vi "Actor Core.vi"(8 "error in":errorcluster, 11 "CoolAppProcess in":refnum<class "CoolAppProcess.lvclass">) -> (0 "error out":errorcluster, 3 "Actor out":refnum<class "Actor.lvclass">)   [LabVIEW 2020, in "LAF2024Q2.lvlib" / "CoolAppProcess.lvclass"]
doc: "(<B>Filename</B>: Actor Framework.lvlib:Actor.lvclass:Actor Core.vi)\n\nReceives messages to the actor, reacts to them, and initiates any error handling that may shut the actor down.\n\nDescendant classes may override this VI to append parallel tasks for the actor to complete while it handles messages. Overrides use the Call Parent Class Method node."
uses:
  CoolAppProcess.lvclass
  C:/Program Files (x86)/National Instruments/LabVIEW 2020/vi.lib/ActorFramework/Actor/Actor.lvclass
  <vilib>/ActorFramework/Actor/Actor.lvclass
  Process State.ctl
  f1630098-5edb-487b-b4df-28bc80a2edd7.vi
  LAF2024Q2.lvlib
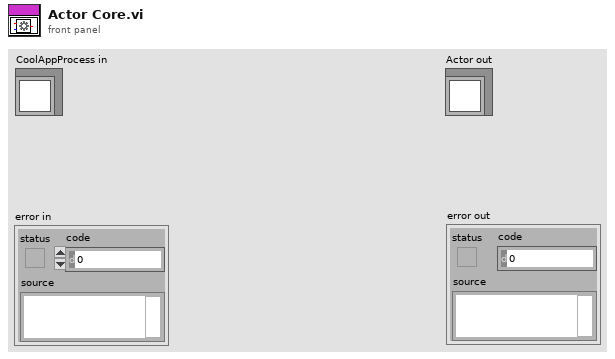
[diagram p1: front panel]
types:
  T1 = typedef "LAF2024Q2.lvlib/Process State.ctl" = enum16{"Idle", "Initializing", "Starting", "Running", "Stopping", "Stopped"}
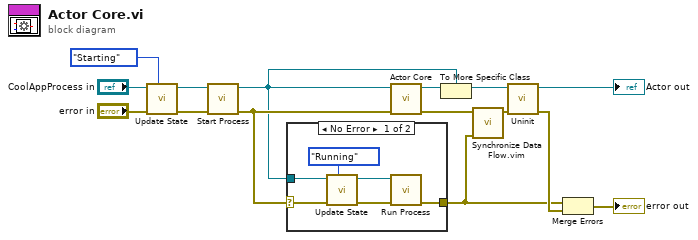
[diagram p0: block diagram]
diagram:
  n1 = call "Update State.vi"("Process State"=Process_State."Starting", "CoolAppProcess in"="CoolAppProcess in") -> ("CoolAppProcess out"=w5:refnum<class "CoolAppProcess.lvclass">)  [unwired: 9 in]
  n2 = call-dynamic "Start Process.vi"("error in (no error)"="error in", "CoolAppProcess in"=w5) -> ("error out"=w7:errorcluster, "CoolAppProcess out"=w6:refnum<class "CoolAppProcess.lvclass">)  [unwired: 8 in]
  n3 = case shown="No Error" w7 {
    selector: w7 -> [w19 _]
    tunnel: w6 -> [w18 _]
    tunnel: [w17 _] -> w1
    frame No Error {
      n4 = call "Update State.vi"("Process State"=Process_State."Running", "CoolAppProcess in"=w18) -> ("CoolAppProcess out"=w16:refnum<class "CoolAppProcess.lvclass">)  [unwired: 9 in]
      n5 = call-dynamic "Run Process.vi"("error in (no error)"=w19, "CoolAppProcess in"=w16) -> ("error out"=w17:errorcluster)  [unwired: 8 in, 1 out]
    }
    frame Error {
    }
  }
  n6 = call-parent "Actor Core.vi"("error in"=w7, "Actor in"=w6) -> ("error out"=w3:errorcluster, "Actor out"=w13:refnum<class "Actor.lvclass">)  [unwired: 8 in]
  n7 = To More Specific Class(target class=w6, reference=w13) -> (specific class reference=w11:refnum<class "CoolAppProcess.lvclass">)  [unwired: 1 in, 1 out]
  n8 = call "Synchronize Data Flow.vim"("input 4"=w1, "input 1"=w3) -> ("output 1"=w2:errorcluster)  [unwired: 2 in, 3 out]
  n9 = call "Uninit.vi"("error in (no error)"=w2, "CoolAppProcess in"=w11) -> ("error out"=w12:errorcluster, "CoolAppProcess out"=→"Actor out":refnum<class "CoolAppProcess.lvclass">)  [unwired: 8 in]
  n10 = Merge Errors(w1, w12) -> (→"error out":errorcluster)
